vi "sensor térmico.vi"(8 "error in (no error)":errorcluster, 10 "noise_gain":dbl=1.0, 11 "dimension size":i32) -> (0 "error out":errorcluster, 3 "Array":dbl[](array[numeric]))   [LabVIEW 2019]
panel:
  in  "Tab Control":enum32{"Page 1", "Page 2"}(tab)
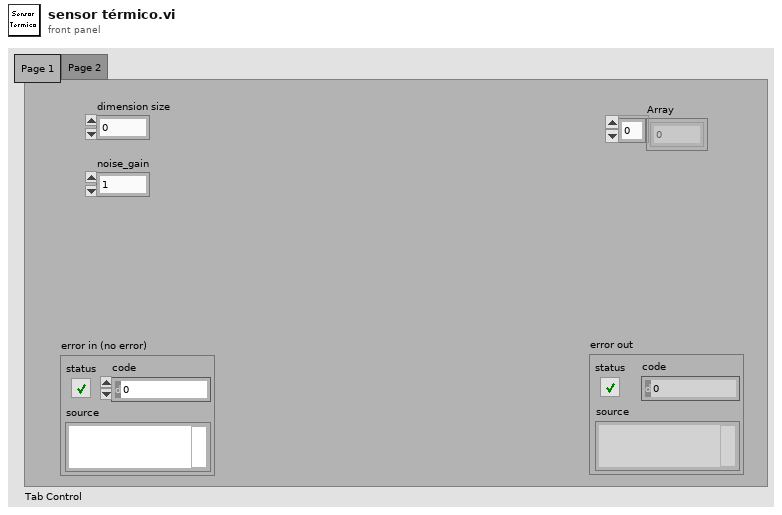
[diagram p1: front panel]
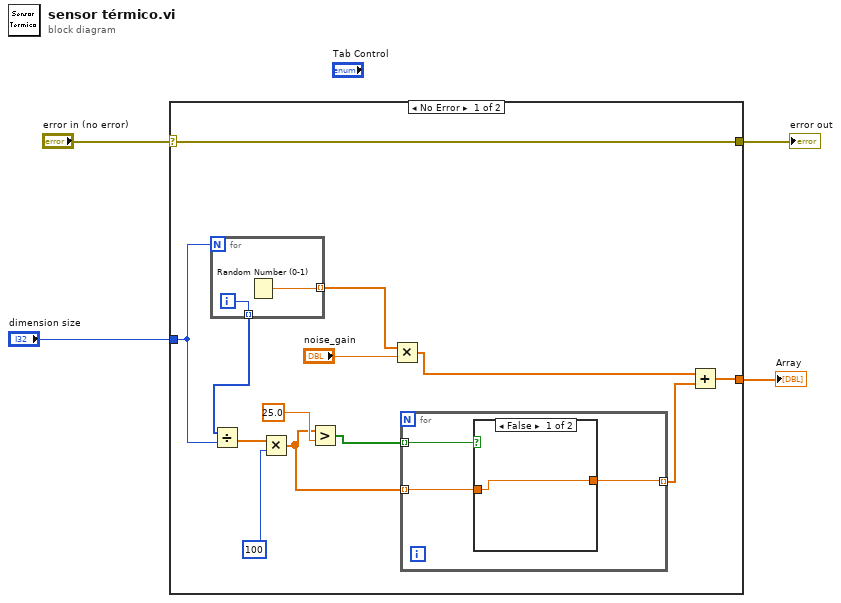
[diagram p0: block diagram]
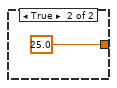
[diagram p2: hidden frame]
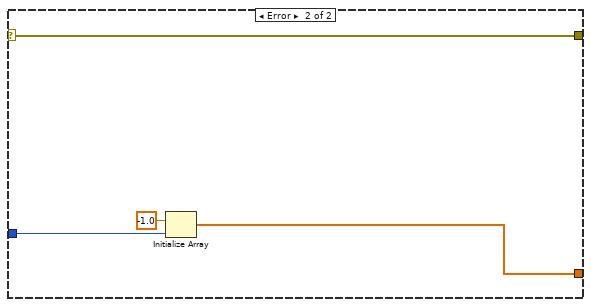
[diagram p3: hidden frame]
diagram:
  n1 = case shown="No Error" "error in (no error)" {
    selector: "error in (no error)" -> [w9 w28]
    tunnel: "dimension size" -> [w15 w27]
    tunnel: [w12 w25] -> w3
    tunnel: [w9 w28] -> w1
    frame No Error {
      n2 = for {
        N: w15 -> [_]
        tunnel: [w24] -> w13 mode=indexing
        tunnel: [w23] -> w14 mode=indexing
        i -> [w23]
        n3 = Random Number (0-1)() -> (number: 0 to 1=w24:dbl)
      }
      n4 = Divide(x=w14, y=w15) -> (x/y=w16:dbl[])
      n5 = Multiply(x=w16, y=100) -> (x*y=w7:dbl[])
      n6 = Greater?(x=w7, y=25.0) -> (0:w6:bool[])
      n7 = Multiply(x=w13, y="noise_gain") -> (x*y=w10:dbl[])
      n8 = for {
        tunnel: w7 -> [w18] mode=indexing
        tunnel: w6 -> [w20] mode=indexing
        tunnel: [w19] -> w5 mode=indexing
        n9 = case shown="False" w20 {
          tunnel: [w21 25.0] -> w19
          tunnel: w18 -> [w21 _]
          frame False {
          }
          frame True {
          }
        }
      }
      n10 = Add(x=w10, y=w5) -> (x+y=w12:dbl[])
    }
    frame Error {
      n11 = Initialize Array(-1.0 ("element"), w27) -> (w25:dbl[])
    }
  }
  "Array" <- w3
  "error out" <- w1
